vi "Actor Core.vi"(8 "error in":cluster{"状态":bool, "代码":i32, "源":string} caption="错误输入", 11 "蒸发冷却器":refnum<class "Evaporative Cooler.lvclass">) -> (0 "error out":cluster{"状态":bool, "代码":i32, "源":string} caption="错误输出", 3 "操作者输出":refnum<class "Actor.lvclass">)   [LabVIEW 2013, in "Evaporative Cooler.lvlib" / "Evaporative Cooler.lvclass"]
doc: "Actor Core.vi包含操作者的主要消息处理循环。操作者通常位于该循环中，在各种消息到达时对消息进行处理。如Do.vi消息返回任何错误，该循环将停止运行，错误代码43将被作为“无错误停止”的标准信号发送给调用方。如需更改上述行为，可在子孙类的Handle Error.vi中对该部分逻辑进行重写。"
uses:
  Evaporative Cooler.lvclass
  <vilib>/ActorFramework/Actor/Actor.lvclass
  Cooler Update Fan Status Msg/Cooler Update Fan Status Msg.lvclass
  Cooler Update Water Level Msg/Cooler Update Water Level Msg.lvclass
  <vilib>/ActorFramework/Actor/Actor.lvclass/Actor.ctl
  <vilib>/ActorFramework/Message Enqueuer/Message Enqueuer.lvclass/Message Enqueuer.ctl
  Timed Loop Actor/Timed Loop Actor/Timed Loop Actor.lvclass/Timed Loop Actor.ctl
  Dual Fan/Dual Fan/Dual Fan.lvclass/Dual Fan.ctl
  Water Level/Water Level.lvclass/Water Level.ctl
  Evaporative Cooler.lvclass/Evaporative Cooler.ctl
  Cooler/Cooler/Cooler.lvclass
  <vilib>/ActorFramework/Message Enqueuer/Init from Existing Queue.vi
  <vilib>/Utility/LVClass/Get LV Class Path.vi
  <vilib>/ActorFramework/Message Enqueuer/Message Enqueuer.lvclass
  Dual Fan/Dual Fan/Dual Fan.lvclass
  Level Controller/Level Controller/Level Controller.lvclass
  Timed Loop Actor/Timed Loop Actor/Timed Loop Actor.lvclass
  Water Level/Water Level.lvclass
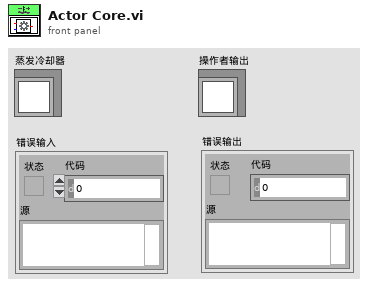
[diagram p1: front panel]
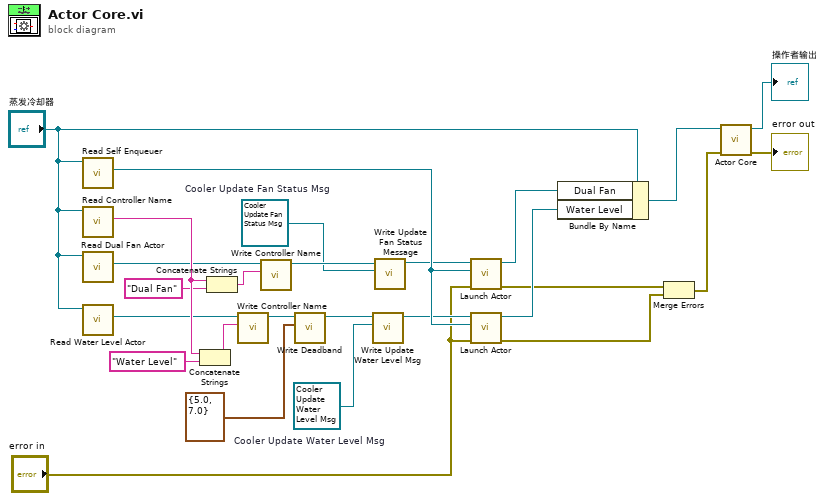
[diagram p0: block diagram]
diagram:
  w2 = refnum<class "Cooler Update Water Level Msg.lvclass"> refnum  # Cooler Update Water Level Msg
  w9 = refnum<class "Cooler Update Fan Status Msg.lvclass"> refnum  # Cooler Update Fan Status Msg
  n1 = call <vilib>:"Read Self Enqueuer.vi"("Actor"="蒸发冷却器") -> ("Self Enqueuer"=w23:refnum<class "Message Enqueuer.lvclass">)  [unwired: 10 in]
  n2 = call "Read Controller Name.vi"("定时循环控制器"="蒸发冷却器") -> ("控制器名称"=w13:string)  [unwired: 10 in]
  n3 = call-dynamic "Read Dual Fan Actor.vi"("蒸发冷却器"="蒸发冷却器") -> ("双风扇"=w8:refnum<class "Dual Fan.lvclass">)  [unwired: 10 in]
  n4 = call-dynamic "Read Water Level Actor.vi"("蒸发冷却器"="蒸发冷却器") -> ("水位"=w6:refnum<class "Water Level.lvclass">)  [unwired: 10 in]
  n5 = Concatenate Strings(w13, "Water Level" ("string")) -> (w14:string)
  n6 = Concatenate Strings(w13, "Dual Fan" ("string")) -> (w10:string)
  n7 = call "Write Controller Name.vi"("控制器名称"=w14, "定时循环控制器输入"=w6) -> ("定时循环控制器输出"=w5:refnum<class "Water Level.lvclass">)  [unwired: 9 in]
  n8 = call "Write Controller Name.vi"("控制器名称"=w10, "定时循环控制器输入"=w8) -> ("定时循环控制器输出"=w15:refnum<class "Dual Fan.lvclass">)  [unwired: 9 in]
  n9 = call "Write Deadband.vi"("死区"=cluster{"LO":dbl, "HI":dbl} {"LO"=5.0, "HI"=7.0} ("Deadband"), "水位控制器输入"=w5) -> ("水位控制器输出"=w4:refnum<class "Water Level.lvclass">)  [unwired: 8 in, 1 out]
  n10 = call "Write Update Water Level Msg.vi"("更新水位消息"=w2, "水位输入"=w4) -> ("水位输出"=w3:refnum<class "Water Level.lvclass">)  [unwired: 9 in]
  n11 = call "Write Update Fan Status Message.vi"("更新消息"=w9, "双风扇输入"=w15) -> ("双风扇输出"=w21:refnum<class "Dual Fan.lvclass">)  [unwired: 9 in]
  n12 = call <vilib>:"Launch Actor.vi"("error in (no error)"="error in", "Actor-to-Caller Enqueuer"=w23, "Actor"=w21) -> ("error out"=w19:errorcluster, "Caller-To-Actor Enqueuer"=w22:refnum<class "Message Enqueuer.lvclass">)  [unwired: 7 in]
  n13 = call <vilib>:"Launch Actor.vi"("error in (no error)"="error in", "Actor-to-Caller Enqueuer"=w23, "Actor"=w3) -> ("error out"=w18:errorcluster, "Caller-To-Actor Enqueuer"=w24:refnum<class "Message Enqueuer.lvclass">)  [unwired: 7 in]
  n14 = Bundle By Name(cluster="蒸发冷却器", "Dual Fan"=w22, "Water Level"=w24) -> (w20:refnum<class "Evaporative Cooler.lvclass">)
  n15 = Merge Errors(w19, w18) -> (w17:errorcluster)
  n16 = call-parent "Actor Core.vi"("error in"=w17, "定时循环控制器"=w20) -> ("error out"=→"error out":cluster{"状态":bool, "代码":i32, "源":string}, "操作者输出"=→"操作者输出":refnum<class "Actor.lvclass">)  [unwired: 8 in]
